vi "chs_to_Netdata.vi"(9 "CHS":T1 {"display" format="%b"}) -> (3 "ChString":string)   [LabVIEW 2011]
uses:
  CHS.ctl
  singlechtype.ctl
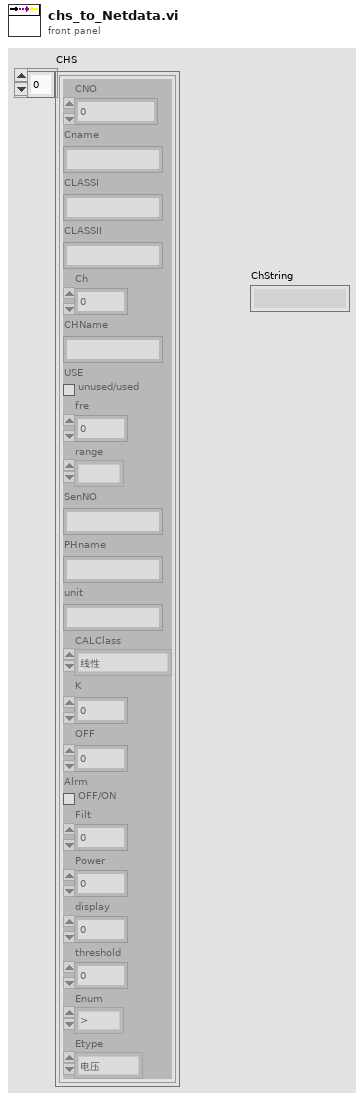
[diagram p1: front panel]
types:
  T1 = typedef "CHS.ctl" = T2[]
  T2 = typedef "singlechtype.ctl" = cluster{"CNO":u8, "Cname":string, "CLASSI":string, "CLASSII":string, "Ch":u8, "CHName":string, "USE":bool, "fre":dbl, "range":enum16{""}, "SenNO":string, "PHname":string, "unit":string, "CALClass":enum8{"线性", "查表", "公式"}, "K":dbl, "OFF":dbl, "Alrm":bool, "Filt":dbl, "Power":u8, "display":u8, "threshold ":dbl, "Enum":enum16{">", ">=", "<", "<=", "<>(在范围内）", "><（在范围外）"}, "Etype":enum16{"电压", "电流", "电阻", "热电偶K", "热电偶T"}}
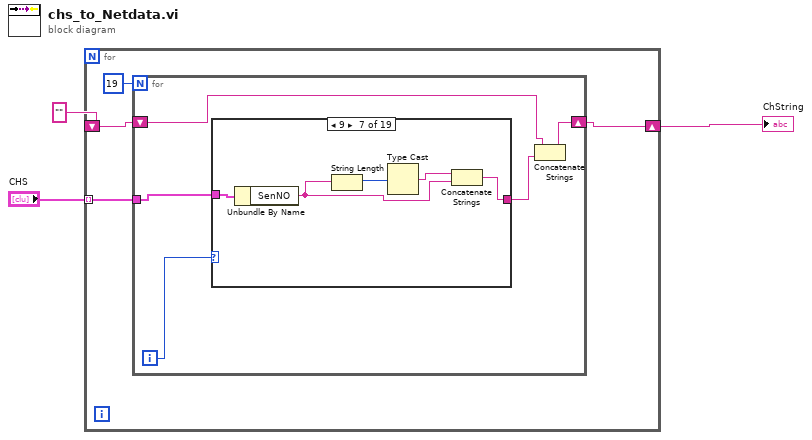
[diagram p0: block diagram]
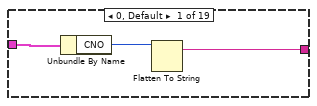
[diagram p2: hidden frame]
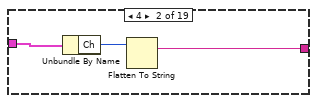
[diagram p3: hidden frame]
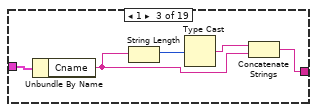
[diagram p4: hidden frame]
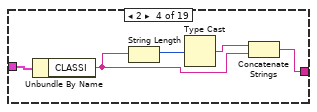
[diagram p5: hidden frame]
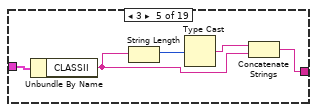
[diagram p6: hidden frame]
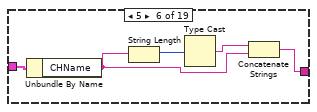
[diagram p7: hidden frame]
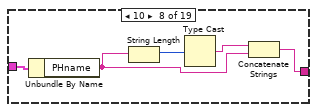
[diagram p8: hidden frame]
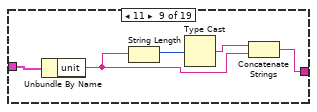
[diagram p9: hidden frame]
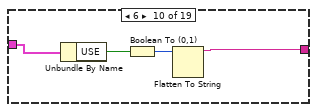
[diagram p10: hidden frame]
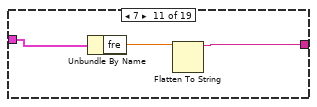
[diagram p11: hidden frame]
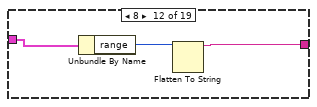
[diagram p12: hidden frame]
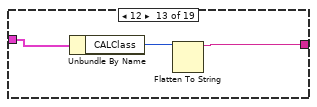
[diagram p13: hidden frame]
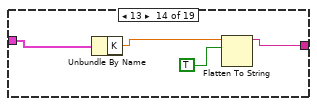
[diagram p14: hidden frame]
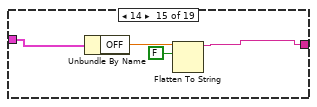
[diagram p15: hidden frame]
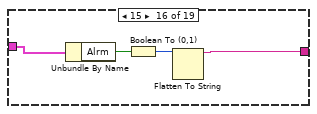
[diagram p16: hidden frame]
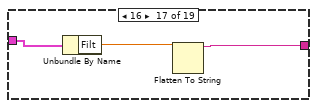
[diagram p17: hidden frame]
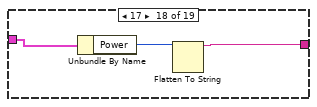
[diagram p18: hidden frame]
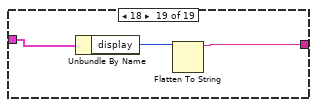
[diagram p19: hidden frame]
diagram:
  n1 = for {
    tunnel: "CHS" -> [w7] mode=indexing
    shift-right: [w5] -> w1
    shift-left: "" -> [w6]
    n2 = for {
      N: 19 -> [_]
      tunnel: w7 -> [w11]
      shift-right: [w8] -> w5
      shift-left: w6 -> [w10]
      i -> [w12]
      n3 = case shown="9" w12 {
        tunnel: w11 -> [w15 w18 w19 w24 w29 w34 w39 w44 w49 w56 w58 w61 w64 w68 w74 w76 w79 w82 w85]
        tunnel: [w13 w16 w20 w25 w30 w35 w40 w45 w50 w55 w59 w62 w65 w69 w71 w77 w80 w83 w86] -> w9
        frame 0, Default {
          n4 = Unbundle By Name(w15) -> ("CNO"=w14:u8)
          n5 = Flatten To String(anything=w14) -> (data string=w13:string)  [unwired: 3 in, 2 out]
        }
        frame 4 {
          n6 = Unbundle By Name(w18) -> ("Ch"=w17:u8)
          n7 = Flatten To String(anything=w17) -> (data string=w16:string)  [unwired: 3 in, 2 out]
        }
        frame 1 {
          n8 = Unbundle By Name(w19) -> ("Cname"=w21:string)
          n9 = String Length(string=w21) -> (length=w23:i32)
          n10 = Type Cast(x=w23) -> (*(type *) &x=w22:string)  [unwired: 1 in]
          n11 = Concatenate Strings(w22, w21) -> (w20:string)
        }
        frame 2 {
          n12 = Unbundle By Name(w24) -> ("CLASSI"=w26:string)
          n13 = String Length(string=w26) -> (length=w28:i32)
          n14 = Type Cast(x=w28) -> (*(type *) &x=w27:string)  [unwired: 1 in]
          n15 = Concatenate Strings(w27, w26) -> (w25:string)
        }
        frame 3 {
          n16 = Unbundle By Name(w29) -> ("CLASSII"=w31:string)
          n17 = String Length(string=w31) -> (length=w33:i32)
          n18 = Type Cast(x=w33) -> (*(type *) &x=w32:string)  [unwired: 1 in]
          n19 = Concatenate Strings(w32, w31) -> (w30:string)
        }
        frame 5 {
          n20 = Unbundle By Name(w34) -> ("CHName"=w36:string)
          n21 = String Length(string=w36) -> (length=w38:i32)
          n22 = Type Cast(x=w38) -> (*(type *) &x=w37:string)  [unwired: 1 in]
          n23 = Concatenate Strings(w37, w36) -> (w35:string)
        }
        frame 9 {
          n24 = Unbundle By Name(w39) -> ("SenNO"=w41:string)
          n25 = String Length(string=w41) -> (length=w43:i32)
          n26 = Type Cast(x=w43) -> (*(type *) &x=w42:string)  [unwired: 1 in]
          n27 = Concatenate Strings(w42, w41) -> (w40:string)
        }
        frame 10 {
          n28 = Unbundle By Name(w44) -> ("PHname"=w46:string)
          n29 = String Length(string=w46) -> (length=w48:i32)
          n30 = Type Cast(x=w48) -> (*(type *) &x=w47:string)  [unwired: 1 in]
          n31 = Concatenate Strings(w47, w46) -> (w45:string)
        }
        frame 11 {
          n32 = Unbundle By Name(w49) -> ("unit"=w51:string)
          n33 = String Length(string=w51) -> (length=w53:i32)
          n34 = Type Cast(x=w53) -> (*(type *) &x=w52:string)  [unwired: 1 in]
          n35 = Concatenate Strings(w52, w51) -> (w50:string)
        }
        frame 6 {
          n36 = Unbundle By Name(w56) -> ("USE"=w57:bool)
          n37 = Boolean To (0,1)(Boolean=w57) -> (0, 1=w54:i16)
          n38 = Flatten To String(anything=w54) -> (data string=w55:string)  [unwired: 3 in, 2 out]
        }
        frame 7 {
          n39 = Unbundle By Name(w58) -> ("fre"=w60:dbl)
          n40 = Flatten To String(anything=w60) -> (data string=w59:string)  [unwired: 3 in, 2 out]
        }
        frame 8 {
          n41 = Unbundle By Name(w61) -> ("range"=w63:enum16{""})
          n42 = Flatten To String(anything=w63) -> (data string=w62:string)  [unwired: 3 in, 2 out]
        }
        frame 12 {
          n43 = Unbundle By Name(w64) -> ("CALClass"=w66:enum8{"线性", "查表", "公式"})
          n44 = Flatten To String(anything=w66) -> (data string=w65:string)  [unwired: 3 in, 2 out]
        }
        frame 13 {
          n45 = Unbundle By Name(w68) -> ("K"=w70:dbl)
          n46 = Flatten To String(anything=w70, prepend array or string size? (T)=TRUE) -> (data string=w69:string)  [unwired: 2 in, 2 out]
        }
        frame 14 {
          n47 = Unbundle By Name(w74) -> ("OFF"=w72:dbl)
          n48 = Flatten To String(anything=w72, prepend array or string size? (T)=FALSE) -> (data string=w71:string)  [unwired: 2 in, 2 out]
        }
        frame 15 {
          n49 = Unbundle By Name(w76) -> ("Alrm"=w78:bool)
          n50 = Boolean To (0,1)(Boolean=w78) -> (0, 1=w75:i16)
          n51 = Flatten To String(anything=w75) -> (data string=w77:string)  [unwired: 3 in, 2 out]
        }
        frame 16 {
          n52 = Unbundle By Name(w79) -> ("Filt"=w81:dbl)
          n53 = Flatten To String(anything=w81) -> (data string=w80:string)  [unwired: 3 in, 2 out]
        }
        frame 17 {
          n54 = Unbundle By Name(w82) -> ("Power"=w84:u8)
          n55 = Flatten To String(anything=w84) -> (data string=w83:string)  [unwired: 3 in, 2 out]
        }
        frame 18 {
          n56 = Unbundle By Name(w85) -> ("display"=w87:u8)
          n57 = Flatten To String(anything=w87) -> (data string=w86:string)  [unwired: 3 in, 2 out]
        }
      }
      n58 = Concatenate Strings(w10, w9) -> (w8:string)
    }
  }
  "ChString" <- w1
